vi "SaveData Data.vi"() -> (0 "SavaData Data":T1={"Configuration"={"Workspace Info"={"Device Name"="ProberHead_Tst_C29K3_7(2)", "Device Info"="ProberHead_Tst_C29", "Path"=path "C:/Users/gio/Desktop/ProbeHeadTest"}, "Instrument Configuration"={"Instrument"=enum."Switching Matrix", "Configuration"="Test Configuration"}, "Stress Motor Position"=0.0, "Electrical Measurement"={"Sequence"=[], "V1"=[], "V2"=[], "V3"=[], "V4"=[], "I1"=[], "I2"=[], "I3"=[], "I4"=[]}, "Optical Spectrum"={"Intensity"=[], "Wavelength"=[], "Energy"=[], "Raman Shift"=[], "Detector Temperature"=0.0}}, "Initialization"={"Start Python Session"=FALSE, "Set Datastructures to Default"=FALSE}})   [LabVIEW 2014]
uses:
  SaveData Data.ctl
  SaveData Config.ctl
  SaveData Workspace Info.ctl
  SaveData Instrument Configuration.ctl
  Instrument Sequence/Instrument List.ctl
  Hardware Control/Spectrometer/Spectral Data.ctl
  SaveData Initialization.ctl
panel:
  # "LICENSED MATERIALS – PROPERTY OF IBM\nCopyright IBM Corp. 2016,\nALL RIGHTS RESERVED"
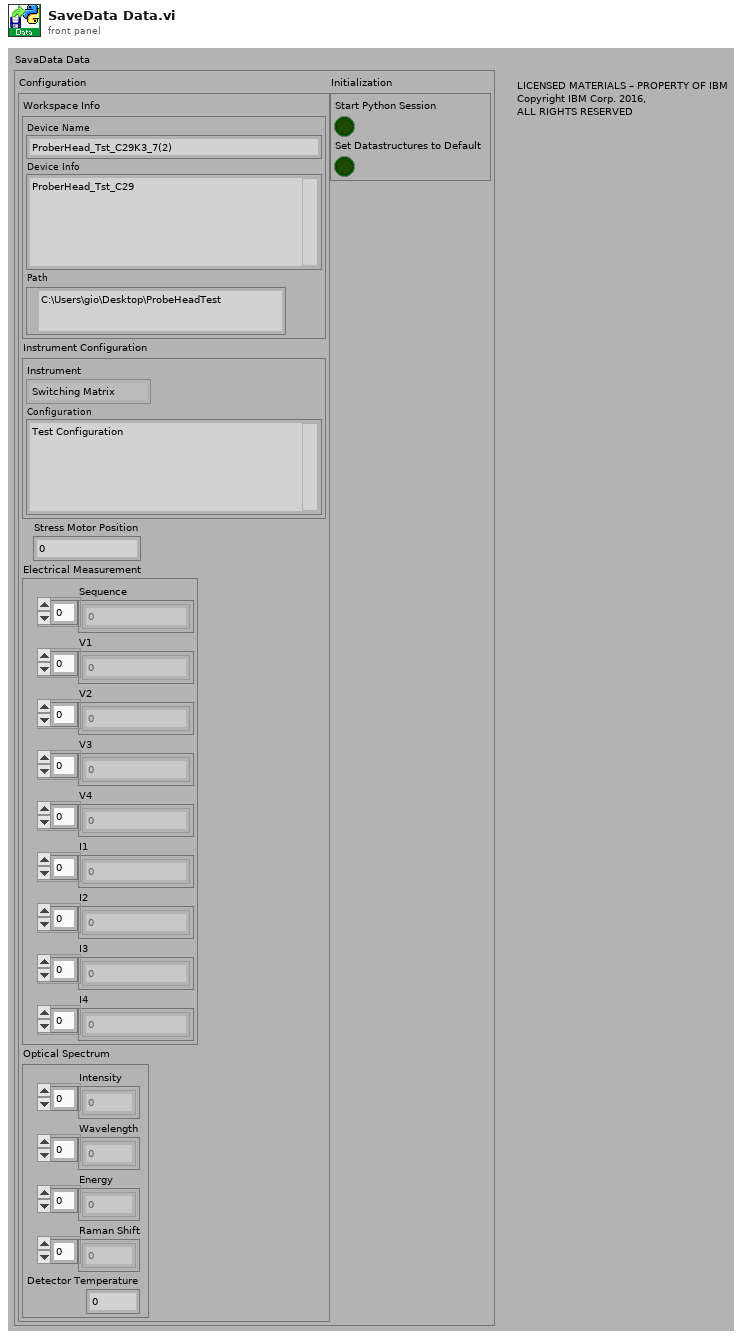
[diagram p1: front panel]
types:
  T1 = typedef "SaveData Data.ctl" = cluster{"Configuration":T2, "Initialization":T7}
  T2 = typedef "SaveData Config.ctl" = cluster{"Workspace Info":T3, "Instrument Configuration":T4, "Stress Motor Position":dbl, "Electrical Measurement":cluster{"Sequence":dbl[], "V1":dbl[], "V2":dbl[], "V3":dbl[], "V4":dbl[], "I1":dbl[], "I2":dbl[], "I3":dbl[], "I4":dbl[]}, "Optical Spectrum":T6}
  T3 = typedef "SaveData Workspace Info.ctl" = cluster{"Device Name":string, "Device Info":string, "Path":path}
  T4 = typedef "SaveData Instrument Configuration.ctl" = cluster{"Instrument":T5, "Configuration":string}
  T5 = typedef "Instrument List.ctl" = enum32{"Unknown Instrument", "Switching Matrix", "Parameter Analyzer", "Optical Spectrometer", "Optoelectronic", "Autofocus"}
  T6 = typedef "Spectral Data.ctl" = cluster{"Intensity":dbl[], "Wavelength":dbl[], "Energy":dbl[], "Raman Shift":dbl[], "Detector Temperature":dbl}
  T7 = typedef "SaveData Initialization.ctl" = cluster{"Start Python Session":bool, "Set Datastructures to Default":bool}
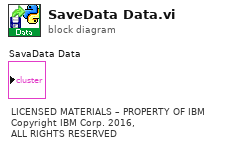
[diagram p0: block diagram]
diagram:
  # "LICENSED MATERIALS – PROPERTY OF IBM\nCopyright IBM Corp. 2016,\nALL RIGHTS RESERVED"
